vi "save_images.vi"(7 "save recorded images":bool, 10 "p_experiment_path":path, 11 "number of fringes":dbl=4.0) -> ()   [LabVIEW 2011]
uses:
  global_vars.vi
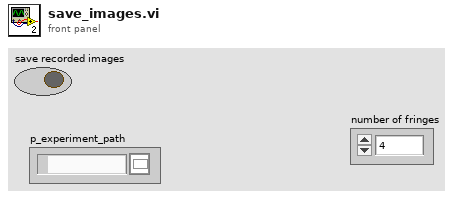
[diagram p1: front panel]
types:
  T1 = typedef "Image Type" = u32
  T2 = typedef "IMAQ Image.ctl" = refnum<image>
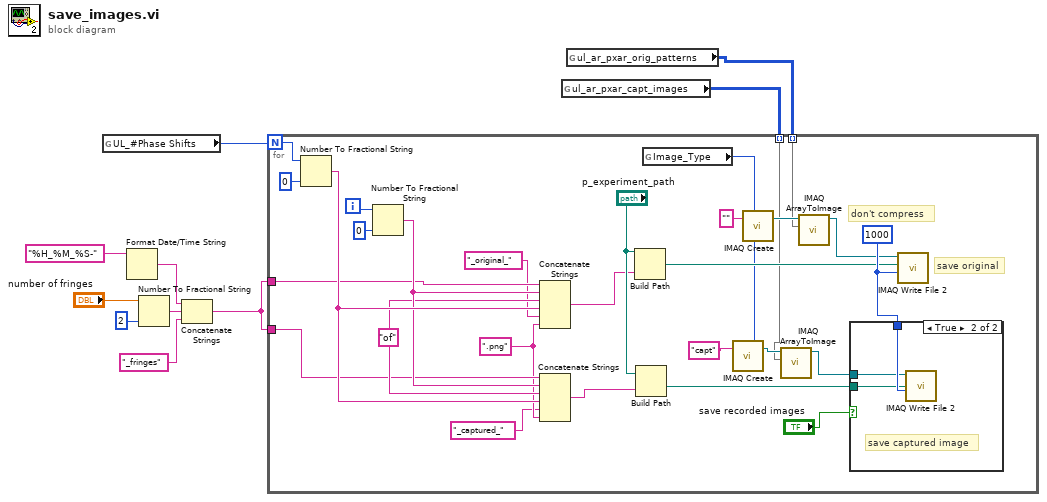
[diagram p0: block diagram]
diagram:
  n1 = global read "global_vars.vi" "UL_#Phase Shifts"() -> (w4:i32)
  n2 = Format Date/Time String(time format string (%c)="%H_%M_%S-") -> (date/time string=w9:string)  [unwired: 2 in]
  n3 = Number To Fractional String(number="number of fringes", precision (6)=i16 2) -> (F-format string=w8:string)  [unwired: 2 in]
  n4 = Concatenate Strings(w9, w8, "_fringes" ("string")) -> (w3:string)
  n5 = global read "global_vars.vi" "ul_ar_pxar_capt_images"() -> (w1:u8[][][])
  n6 = global read "global_vars.vi" "ul_ar_pxar_orig_patterns"() -> (w2:u8[][][])
  n7 = for {
    N: w4 -> [w34]
    tunnel: w3 -> [w27]
    tunnel: w3 -> [w24]
    tunnel: w2 -> [w11] mode=indexing
    tunnel: w1 -> [w12] mode=indexing
    i -> [w30]
    w23 = ".png" ("string")
    w28 = "of" ("string")
    w38 = u32 1000 ("Image Quality")
    # "don't compress"
    # "save original"
    n8 = Number To Fractional String(number=w34, precision (6)=i16 0) -> (F-format string=w32:string)  [unwired: 2 in]
    n9 = Number To Fractional String(number=w30, precision (6)=i16 0) -> (F-format string=w29:string)  [unwired: 2 in]
    n10 = Concatenate Strings(w27, w29, w28, w32, "_original_" ("name or relative path"), w23) -> (w26:string)
    n11 = Concatenate Strings(w24, w29, w28, w32, "_captured_" ("name or relative path"), w23) -> (w25:string)
    n12 = Build Path(base path="p_experiment_path", name or relative path=w26) -> (appended path=w35:path)
    n13 = Build Path(base path="p_experiment_path", name or relative path=w25) -> (appended path=w36:path)
    n14 = global read "global_vars.vi" "Image_Type"() -> (w13:T1)
    n15 = call "IMAQ Create"("Image Name"="capt", "Image Type"=w13) -> ("New Image"=w19:T2)  [unwired: 2 in, 2 out]
    n16 = call "IMAQ Create"("Image Name"="", "Image Type"=w13) -> ("New Image"=w15:T2)  [unwired: 2 in, 2 out]
    n17 = call "IMAQ ArrayToImage"("Image Pixels (U8)"=w12, "Image"=w19) -> ("Image Out"=w21:T2)  [unwired: 8 in, 1 out]
    n18 = call "IMAQ ArrayToImage"("Image Pixels (U8)"=w11, "Image"=w15) -> ("Image Out"=w20:T2)  [unwired: 8 in, 1 out]
    n19 = case shown="True" "save recorded images" {
      tunnel: w38 -> [_ w41]
      tunnel: w36 -> [_ w40]
      tunnel: w21 -> [_ w39]
      frame False {
      }
      frame True {
        # "save captured image"
        n20 = call-poly "IMAQ Write File 2"("Image Quality"=w41, "File Path"=w40, "Image"=w39) -> ()  [unwired: 7 in, 2 out]
      }
    }
    n21 = call-poly "IMAQ Write File 2"("Image Quality"=w38, "File Path"=w35, "Image"=w20) -> ()  [unwired: 7 in, 2 out]
  }
